vi "msg.self_lua.vi"(5 "LuaVIEW reference":T1) -> (15 "error out":errorcluster)   [LabVIEW 2012]
doc: "Have a task send a message to itself. This can help simplify a task's implementation by removing the need for special-casing the handling of self-initiated actions.\nParameters:\nstr:message\nErrors:\nFunction must be called from a task context but was not."
uses:
  typedefs/t_LuaVIEW Reference.ctl
  typedefs/t_LuaVIEW Task State Methods.ctl
  subvis/private/LuaVIEW Pull (string).vi
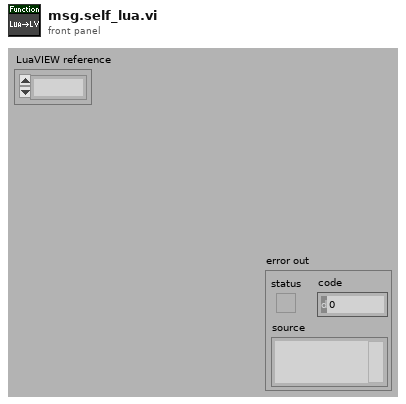
[diagram p1: front panel]
types:
  T1 = typedef "t_LuaVIEW Reference.ctl" = refnum<k1>
  T2 = typedef "t_LuaVIEW Task State Methods.ctl" = enum16{"cleanup", "set initial", "set mode", "set active mode", "set error", "get task info", "get script info", "set signal", "clear signal", "test handled", "test delegated", "test signal", "handle signal", "delegate signal", "allow signal", "disallow signal", "disallow all", "signals?", "delegated signals?", "protection++", "protection--", "protection=0", "message", "next message", "pop message", "message available?", "force stop", "set swap preps", "apply swap preps"}
  T3 = typedef "t_LuaVIEW Task State Pane.ctl" = refnum<vi>
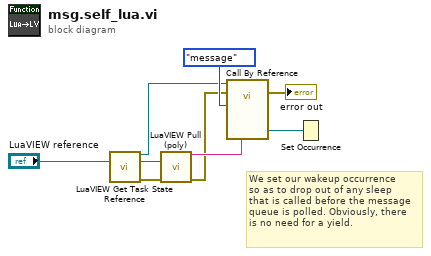
[diagram p0: block diagram]
diagram:
  # "We set our wakeup occurrence\nso as to drop out of any sleep\nthat is called before the message\nqueue is polled. Obviously, there\nis no need for a yield."
  n1 = call "LuaVIEW Get Task State Reference.vi"("LuaVIEW reference in"="LuaVIEW reference") -> ("task state reference"=w2:T3, "LuaVIEW reference out"=w4:T1, "error out"=w5:errorcluster)  [unwired: 12 in]
  n2 = call-poly "LuaVIEW Pull (poly).vi"("LuaVIEW reference in"=w4, "error in (no error)"=w5) -> ("string"=w7:string, "error out"=w6:errorcluster)  [unwired: 11 in, 1 out]
  n3 = call-by-ref "?"(reference=w2, error in=w6, "method"=t_LuaVIEW_Task_State_Methods."message", "string in"=w7) -> (error out=→"error out":errorcluster, "wakeup occurrence"=w1:refnum<k4>)  [unwired: 9 in, 5 out]
  n4 = Set Occurrence(w1) -> ()
